vi "IRSensorNIRead.vi"(8 "error in (no error)":errorcluster, 9 "Melexis_Cmmds":u8(ring)=46 format="%08b" items=["RAM IR raw  Ch1"=4, "RAM IR raw  Ch2"=5, "RAM T_A"=6, "RAM T_OBJ1"=7, "RAM T_OBJ2"=8, "EEPROM_To_max"=32, "EEPROM_To_min"=33, "EEPROM_PWM_CTRL"=34, "EEPROM_Ta_range"=35, "EEPROM_Emissivity_CorrCoeff"=36, "EEPROM_SMBus Address"=46, "EEPROM_ConfigReg"=37], 10 "Address":u8=80 format="%.0x", 11 "device reference":T1) -> (0 "error out":errorcluster, 2 "Temperature":dbl, 3 "device reference out":T1)   [LabVIEW 2015]
uses:
  <vilib>/ni845x/ni845x.llb/ni845xControl.ctl
  <vilib>/ni845x/ni845x.llb/ni845xI2cConfiguration.ctl
  <resource>/objmgr/NI845x.rc
panel:
  out "appended array":u8[](array[numeric])
  out "i2c configuration out":T2
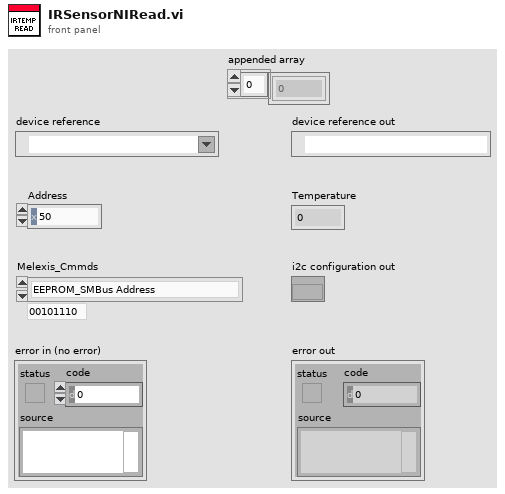
[diagram p1: front panel]
types:
  T1 = typedef "ni845xControl.ctl" = refnum<k21>
  T2 = typedef "ni845xI2cConfiguration.ctl" = refnum<k20>
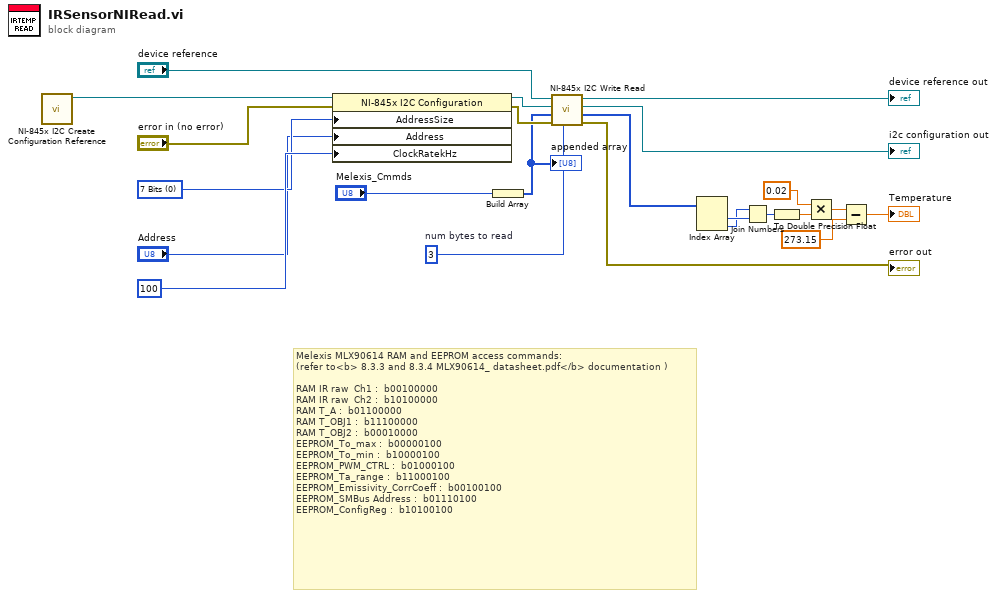
[diagram p0: block diagram]
diagram:
  w14 = u32 3  # num bytes to read
  w20 = 0 items=["7 Bits", "10 Bits"] ("Address Size")
  # "Melexis MLX90614 RAM and EEPROM access commands:\n(refer to<b> 8.3.3 and 8.3.4 MLX90614_ datasheet.pdf</b> documentation )\n\nRAM IR raw  Ch1 :  b00100000\nRAM IR raw  Ch2 :  b10100000\nRAM T_A :  b01100000\nRAM T_OBJ1 :  b11100000\nRAM T_OBJ2 :  b00010000\nEEPROM_To_max :  b00000100\nEEPROM_To_min :  b10000100\nEEPROM_PWM_CTRL :  b01000100\nEEPROM_Ta_range :  b11000100\nEEPROM_Emissivity_CorrCoeff :  b00100100\nEEPROM_SMBus Address :  b01110100\nEEPROM_ConfigReg :  b10100100"
  n1 = call <vilib>:"NI-845x I2C Create Configuration Reference.vi"() -> ("i2c configuration"=w23:T2)  [unwired: 10 in, 1 out]
  n2 = property class="NI-845x I2C Configuration"(reference=w23, error in="error in (no error)", "AddressSize"=w20, "Address"="Address", "ClockRatekHz"=u16 100 ("Clock Rate in kHz")) -> (reference out=w19:T2, error out=w17:errorcluster)
  n3 = Build Array("Melexis_Cmmds") -> (w15:u8[])
  "appended array" <- w15
  n4 = call <vilib>:"NI-845x I2C Write Read.vi"("num bytes to read"=w14, "error in (no error)"=w17, "write data"=w15, "i2c configuration in"=w19, "device reference in"="device reference") -> ("error out"=→"error out":errorcluster, "read data"=w10:u8[], "i2c configuration out"=→"i2c configuration out":T2, "device reference out"=→"device reference out":T1)  [unwired: 3 in]
  n5 = Index Array(array=w10) -> (element #1=w9:u8, element #2=w8:u8)  [unwired: 2 in]
  n6 = Join Numbers(hi=w8, lo=w9) -> ((hi.lo)=w7:u16)
  n7 = To Double Precision Float(number=w7) -> (double precision float=w6:dbl)
  n8 = Multiply(x=0.02, y=w6) -> (x*y=w4:dbl)
  n9 = Subtract(x=w4, y=273.15) -> (x-y=→"Temperature":dbl)
